vi "ChangeIndicator.vi"(0 "Input":variant) -> (6 "Change":bool=TRUE)   [LabVIEW 2015, in "ECS-Host.lvlib"]
uses:
  ECS-Host.lvlib
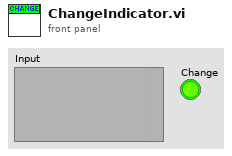
[diagram p1: front panel]
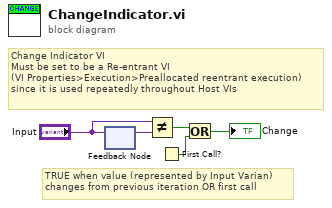
[diagram p0: block diagram]
diagram:
  # "Change Indicator VI\nMust be set to be a Re-entrant VI \n(VI Properties>Execution>Preallocated reentrant execution)\nsince it is used repeatedly throughout Host VIs"
  # "TRUE when value (represented by Input Varian)\nchanges from previous iteration OR first call"
  n1 = feedback-in #1("Input") -> ()
  n2 = feedback #1() -> (w5:variant)  [unwired: 1 in]
  n3 = Not Equal?(x="Input", y=w5) -> (x != y?=w1:bool)
  n4 = First Call?() -> (First Call?: T/F=w2:bool)
  n5 = Or(x=w1, y=w2) -> (x .or. y?=→"Change":bool)
